vi "unpack_bool.vi"(3 "error in":errorcluster, 5 "u":u64) -> (0 "error out":errorcluster, 1 "bool":bool, 2 "u out":u64)   [LabVIEW 2019, in "msgunpack.lvlib"]
doc: "Unpacks a single boolean value from the buffer."
uses:
  msgunpack.lvlib
  msgpack.lvlib
  msgpackalt.dll
panel:
  # "msgpack"
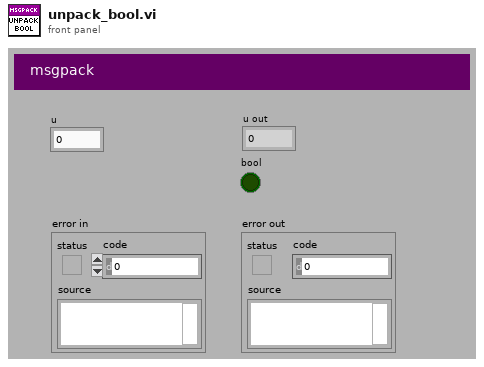
[diagram p1: front panel]
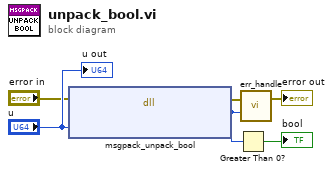
[diagram p0: block diagram]
diagram:
  n1 = dll-call lib="C:/Users/Patrick/Documents/GitHub/Instrument-Framework/lvsrc/SMOs/JSON-RPC-2019/lv-venv/lv.lib/vi.lib/addons/msgpack/msgpackalt.dll" fn="msgpack_unpack_bool"(error in="error in", "p"="u") -> (error out=w4:errorcluster, "return type"=w1:i32)  [unwired: 3 in, 1 out]
  n2 = Greater Than 0?(x=w1) -> (x > 0?=→"bool":bool)
  n3 = call "err_handle.vi"("retval"=w1, "error in"=w4) -> ("error out"=→"error out":errorcluster)  [unwired: 1 in]
  "u out" <- "u"
